vi "ws_www template.vi"(6 "User":T1, 7 "httpRequestID":u32, 8 "error in (no error)":errorcluster, 9 "Template Keys (empty)":T3, 10 "Template (\"\")":string, 11 "DB Connection Ref":T2) -> (3 "HTTP Template Content":string)   [LabVIEW 2011]
uses:
  <vilib>/addons/internet/utils/keyedarr.llb/Keyed Array.ctl
  SI.LIB/ODBC/SQL Controls/Connection Refnum.ctl
  server/database/Users/User Record.ctl
  <vilib>/wsapi/NI_WebServices.lvlib
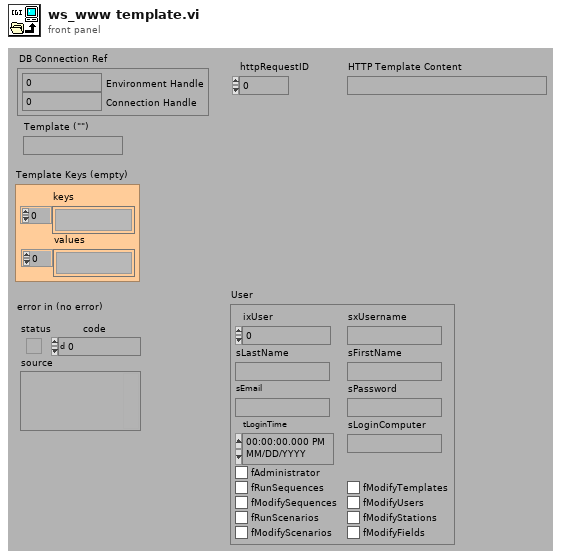
[diagram p1: front panel]
types:
  T1 = typedef "User Record.ctl" = cluster{"ixUser":i32, "sxUsername":string, "sLastName":string, "sFirstName":string, "sEmail":string, "sPassword":string, "tLoginTime":timestamp, "sLoginComputer":string, "fAdministrator":bool, "fRunSequences":bool, "fModifySequences":bool, "fRunScenarios":bool, "fModifyScenarios":bool, "fModifyTemplates":bool, "fModifyUsers":bool, "fModifyStations":bool, "fModifyFields":bool}
  T2 = typedef "Connection Refnum.ctl" = cluster{"Environment Handle":i32, "Connection Handle":i32}
  T3 = typedef "Keyed Array.ctl" = cluster{"keys":string[], "values":string[]}
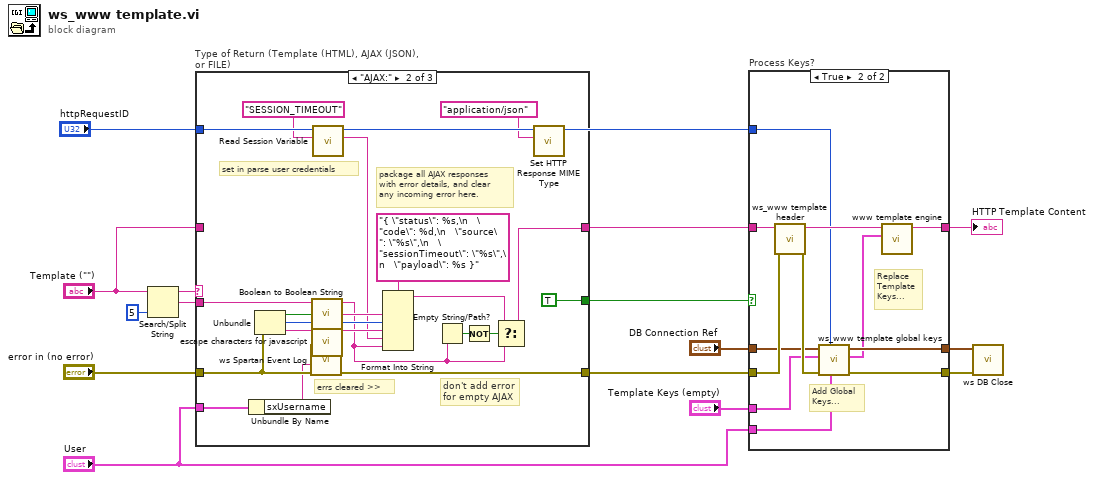
[diagram p0: block diagram]
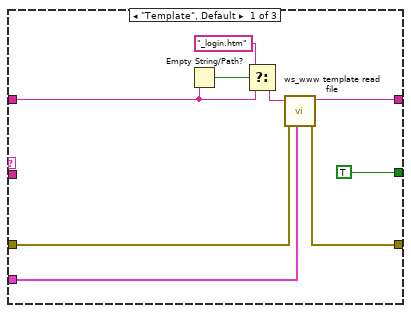
[diagram p3: hidden frame]
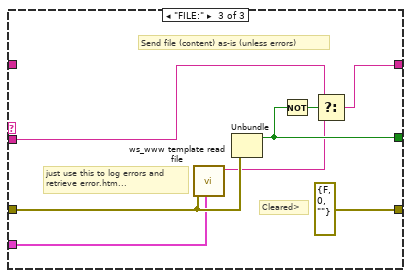
[diagram p4: hidden frame]
diagram:
  n1 = Search/Split String(string="Template (\"\")", offset (0)=5) -> (substring before match=w9:string, match + rest of string=w8:string)  [unwired: 2 out]
  n2 = case "Type of Return (Template (HTML), AJAX (JSON), or FILE)" shown="\"AJAX:\"" w9 {
    tunnel: [w22 w30 errorcluster {"status"=FALSE, "code"=0, "source"=""} ("error out")] -> w13
    tunnel: "error in (no error)" -> [w20 w33 w51]
    tunnel: [w23 w37 w53] -> w11
    tunnel: "User" -> [w21 w31 w46]
    tunnel: w8 -> [_ w35 w47]
    tunnel: [TRUE TRUE w52] -> w7
    tunnel: "Template (\"\")" -> [w17 _ _]
    tunnel: "httpRequestID" -> [_ w29 _]
    frame "Template", Default {
      n3 = Empty String/Path?(string/path=w17) -> (empty?=w19:bool)
      n4 = Select(t="_login.htm" ("Template (\"\")"), s=w19, f=w17) -> (s? t:f=w16:string)
      n5 = call "ws_www template read file.vi"("User"=w21, "error in (no error)"=w20, "Template File (\"\")"=w16) -> ("error out"=w22:errorcluster, "Page HTML"=w23:string)  [unwired: 1 in, 6 out]
    }
    frame "AJAX:" {
      # "set in parse user credentials"
      # "errs cleared >>"
      # "don't add error\nfor empty AJAX"
      # "package all AJAX responses\nwith error details, and clear\nany incoming error here."
      n6 = Unbundle By Name(w31) -> ("sxUsername"=w32:string)
      n7 = Unbundle(w33) -> ("status"=w43:bool, "code"=w42:i32, "source"=w41:string)
      n8 = call "ws Spartan Event Log.vi"("error in (no error)"=w33, "username (\"\")"=w32) -> ("error out"=w30:errorcluster)  [unwired: 6 in]
      n9 = call "Boolean to Boolean String.vi"("Boolean"=w43) -> ("Boolean string"=w44:string)  [unwired: 1 in]
      n10 = call "escape characters for javascript.vi"("String (\"\")"=w41) -> ("escaped String"=w40:string)  [unwired: 4 out]
      n11 = call <vilib>:"Read Session Variable.vi"("key"="SESSION_TIMEOUT", "httpRequestID"=w29) -> ("value"=w27:string, "httpRequestID out"=w26:u32)  [unwired: 7 in, 1 out]
      n12 = Format Into String(format string="{ \"status\": %s,\n   \"code\": %d,\n   \"source\": \"%s\",\n   \"sessionTimeout\": \"%s\",\n   \"payload\": %s }", w44, w42, w40, w27, w35) -> (resulting string=w38:string)  [unwired: 2 in, 1 out]
      n13 = Empty String/Path?(string/path=w35) -> (empty?=w39:bool)
      n14 = Not(x=w39) -> (.not. x?=w36:bool)
      n15 = Select(t=w38, s=w36, f=w35) -> (s? t:f=w37:string)
      n16 = call <vilib>:"Set HTTP Response MIME Type.vi"("MIME type (text/html)"="application/json", "httpRequestID"=w26) -> ()  [unwired: 8 in, 2 out]
    }
    frame "FILE:" {
      # "Cleared>"
      # "just use this to log errors and\nretrieve error.htm..."
      # "Send file (content) as-is (unless errors)"
      n17 = call "ws_www template read file.vi"("User"=w46, "error in (no error)"=w51) -> ("Page HTML"=w49:string)  [unwired: 1 in, 8 out]
      n18 = Unbundle(w51) -> ("status"=w52:bool)  [unwired: 2 out]
      n19 = Not(x=w52) -> (.not. x?=w50:bool)
      n20 = Select(t=w47, s=w50, f=w49) -> (s? t:f=w53:string)
    }
  }
  n21 = case "Process Keys?" shown="True" w7 {
    tunnel: [w55 w68] -> w5
    tunnel: [w56 w67] -> w15
    tunnel: "DB Connection Ref" -> [w54 w61]
    tunnel: [w54 w62] -> w4
    tunnel: w13 -> [w55 w66]
    tunnel: w11 -> [w56 w64]
    tunnel: "httpRequestID" -> [_ w59]
    tunnel: "Template Keys (empty)" -> [_ w58]
    tunnel: "User" -> [_ w57]
    frame False {
    }
    frame True {
      # "Replace\nTemplate\nKeys..."
      # "Add Global\nKeys..."
      n22 = call "ws_www template header.vi"("error in (no error)"=w66, "Template Content (\"\")"=w64) -> ("error out"=w65:errorcluster, "Template Content"=w63:string)  [unwired: 8 in]
      n23 = call "ws_www template global keys.vi"("Current User"=w57, "httpRequestID"=w59, "error in (no error)"=w65, "Template Keys In (empty)"=w58, "DB Connection Ref"=w61) -> ("error out"=w68:errorcluster, "new Template Keys"=w60:T3, "dup DB Connection Ref"=w62:T2)  [unwired: 4 in]
      n24 = call "www template engine.vi"("Template Dictionary (empty)"=w60, "Template String (\"\")"=w63) -> ("Template String out"=w67:string)  [unwired: 1 in, 8 out]
    }
  }
  "HTTP Template Content" <- w15
  n25 = call "ws DB Close.vi"("error in (no error)"=w5, "Connection Refnum"=w4) -> ()  [unwired: 9 in, 1 out]
